vi "Write 1Ch 1Samp (Timestamp).vi"(4 "timestamp":timestamp, 6 "index_channel":u32, 8 "error in":errorcluster, 9 "data":timestamp, 10 "channel":u32, 11 "Writer":refnum<class "Synnax Writer.lvclass">) -> (0 "error out":errorcluster, 3 "Writer Out":refnum<class "Synnax Writer.lvclass">)   [LabVIEW 2026, in "synnax_lib.lvlib" / "Synnax Writer.lvclass"]
uses:
  Synnax Writer.lvclass
  Synnax Writer.lvclass/Synnax Writer.ctl
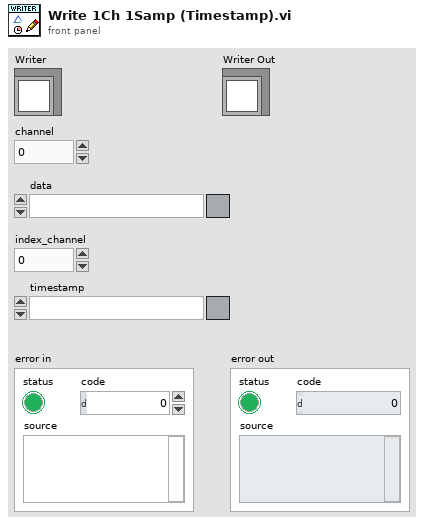
[diagram p1: front panel]
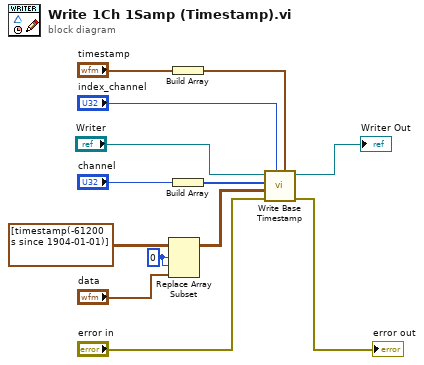
[diagram p0: block diagram]
diagram:
  w5 = 0
  n1 = Replace Array Subset(array=timestamp[][] [timestamp(-61200 s since 1904-01-01)], new element="data", index (row)=w5, index (col)=w5) -> (w3:timestamp[][])
  n2 = Build Array("timestamp") -> (w7:timestamp[])
  n3 = Build Array("channel") -> (w10:u32[])
  n4 = call "Write Base Timestamp.vi"("timestamps"=w7, "index_channel"="index_channel", "error in"="error in", "data"=w3, "channels"=w10, "Writer"="Writer") -> ("error out"=→"error out":errorcluster, "Writer Out"=→"Writer Out":refnum<class "Synnax Writer.lvclass">)  [unwired: 4 in]
